vi "MACBIN Decode MacBinary__ogtk.vi"(4 "error in (no error)":errorcluster, 5 "resource file":path, 6 "data file":path, 7 "macbinary file":path) -> (0 "error out":errorcluster, 1 "resource file out":path, 2 "data file out":path, 3 "macbinary file out":path)   [LabVIEW 2020]
doc: "Decodes a Macintosh File from MacBinary format."
panel:
  # "Please visit http://www.OpenG.org to learn about the\nOpen Source LabVIEW software movement.\n\nNOTICE -- YOU MUST LEAVE THIS NOTICE IN PLACE.  PER THE TERMS OF THE LICENSE BELOW, YOU MAY SUBLICENSE THIS SOFTWARE \nIN ANY WAY THAT DOES NOT CONFLICT WITH THIS LICENSE.\n\n### BSD License (http://www.opensource.org/licenses/bsd-license.php) Begin ###\n \nCopyright (C) 2002 Christophe Salzmann christophe.salzmann@epfl.ch\nCopyright (C) 2002 Rolf Kalbermatter rolf.kalbermatter@citengineering.com\n\nAll rights reserved.\n\nRedistribution and use in source and binary forms, with or without modification, are permitted provided that the following conditions are met:\n\n    * Redistributions of source code must retain the above copyright notice, this list of conditions and the following disclaimer.\n    * Redistributions in binary form must reproduce the above copyright notice, this list of conditions and the following disclaimer in the \n       documentation and/or other materials provided with the distribution.\n    * Neither the name of SciWare, James Kring, Inc., nor the names of its contributors may be used to endorse or promote products derived \n       from this software without specific prior written permission.\n\nTHIS SOFTWARE IS PROVIDED BY THE COPYRIGHT HOLDERS AND CONTRIBUTORS \"AS IS\" AND ANY EXPRESS OR IMPLIED WARRANTIES, \nINCLUDING, BUT NOT LIMITED TO, THE IMPLIED WARRANTIES OF MERCHANTABILITY AND FITNESS FOR A PARTICULAR PURPOSE ARE \nDISCLAIMED. IN NO EVENT SHALL THE COPYRIGHT OWNER OR CONTRIBUTORS BE LIABLE FOR ANY DIRECT, INDIRECT, INCIDENTAL,\n SPECIAL, EXEMPLARY, OR CONSEQUENTIAL DAMAGES (INCLUDING, BUT NOT LIMITED TO, PROCUREMENT OF SUBSTITUTE GOODS OR \nSERVICES; LOSS OF USE, DATA, OR PROFITS; OR BUSINESS INTERRUPTION) HOWEVER CAUSED AND ON ANY THEORY OF LIABILITY, \nWHETHER IN CONTRACT, STRICT LIABILITY, OR TORT (INCLUDING NEGLIGENCE OR OTHERWISE) ARISING IN ANY WAY OUT OF THE USE \nOF THIS SOFTWARE, EVEN IF ADVISED OF THE POSSIBILITY OF SUCH DAMAGE.\n\n### BSD License End ###"
  # "``"
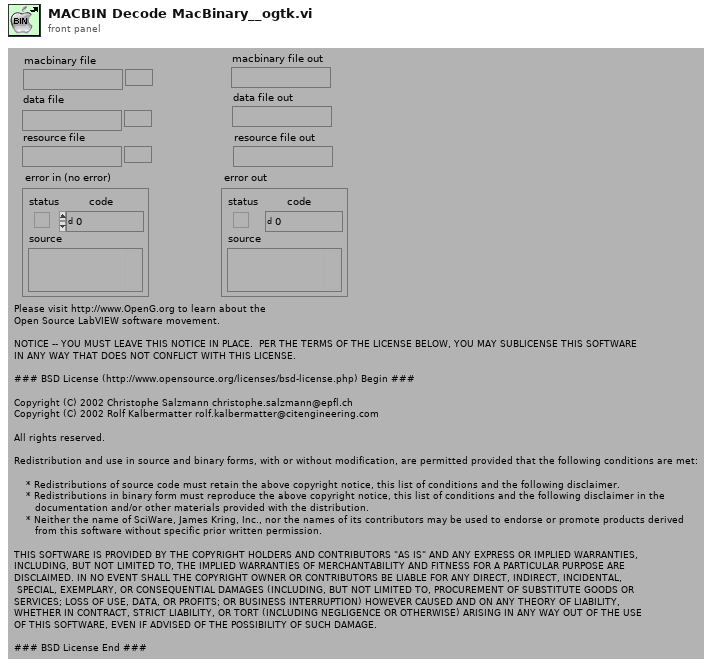
[diagram p1: front panel]
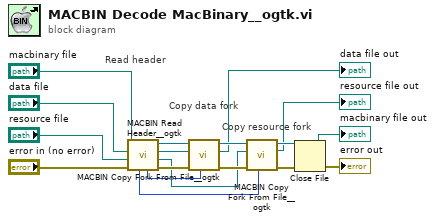
[diagram p0: block diagram]
diagram:
  # "Read header"
  # "Copy resource fork"
  # "Copy data fork"
  n1 = call <userlib>:"MACBIN Read Header__ogtk.vi"("error in (no error)"="error in (no error)", "resource file"="resource file", "data file"="data file", "macbinary file"="macbinary file") -> ("error out"=w14:errorcluster, "res file refnum"=w12:refnum<file>, "data filerefnum"=w13:refnum<file>, "macbin filerefnum"=w10:refnum<file>, "data length"=w9:i32, "res length"=w8:i32)
  n2 = call <userlib>:"MACBIN Copy Fork From File__ogtk.vi"("length"=w9, "error out"=w14, "fork Refnum"=w13, "macbinary Refnum"=w10) -> ("error out"=w17:errorcluster, "forkname out"=→"data file out":path, "macbinary Refnum out"=w16:refnum<file>)  [unwired: 2 in]
  n3 = call <userlib>:"MACBIN Copy Fork From File__ogtk.vi"("length"=w8, "error out"=w17, "fork Refnum"=w12, "macbinary Refnum"=w16) -> ("error out"=w4:errorcluster, "forkname out"=→"resource file out":path, "macbinary Refnum out"=w5:refnum<file>)  [unwired: 2 in]
  n4 = Close File(refnum=w5, error in=w4) -> (path=→"macbinary file out":path, error out=→"error out":errorcluster)
